vi "氨氮测量流程.vi"(11 "控制命令":T1(ring)) -> ()   [LabVIEW 2016, in "斯坦道氨氮.lvlib"]
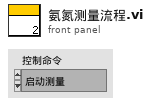
[diagram p1: front panel]
types:
  T1 = enum16{"启动测量", "标样核查", "零点核查", "跨度核查", "空白测试", "平行样测试", "加标回收", "空白校准", "标样校准", "初始化（清洗）", "停止测试", "仪器重启", "校时", "模式设置", "测量间隔设置"}
  T2 = cluster{"时间标识":timestamp, "设备":string, "日志信息":string, "流程参数":string}
  T3 = cluster{"站号":u16, "量程切换":enum32{"H", "L", "AUTO"}, "控制命令":enum16{"启动测量", "标样核查", "零点核查", "跨度核查", "空白测试", "平行样测试", "加标回收", "空白校准", "标样校准", "初始化（清洗）", "停止测试", "仪器重启", "校时", "模式设置", "测量间隔设置"}, "模式设置":enum16{"待机", "连续模式", "周期模式", "定点模式", "受控模式", "手动模式"}, "测量间隔":u16}
  T4 = cluster{"系统时间":timestamp, "工作状态":enum16{"空闲", "水样测试", "标样核查", "零点核查", "跨度核查", "空白测试", "平行样测试", "加标回收", "空白校准", "标样校准", "初始化（清洗）"}, "测量模式":enum16{"待机", "连续模式", "周期模式", "定点模式", "受控模式", "手动模式"}, "告警代码":u16, "故障代码":u16, "日志代码":u16, "软件版本":u16, "F0":sgl, "F1":sgl, "F2":sgl, "F3":sgl, "T":sgl, "H":sgl, "id":u16, "flowid":u16, "量程":u16, "总磷控温温度1":sgl, "营养盐控温温度2":sgl, "ADC":sgl}
  T5 = cluster{"水样测试量程模式":enum16{"H", "L", "AUTO"}, "空白核查量程模式":enum16{"H", "L", "AUTO"}, "跨度核查量程模式":enum16{"H", "L", "AUTO"}, "加标回收量程模式":enum16{"H", "L", "AUTO"}}
  T6 = enum16{"空闲", "水样测试", "标样核查", "零点核查", "跨度核查", "空白测试", "平行样测试", "加标回收", "空白校准", "标样校准", "初始化（清洗）"}
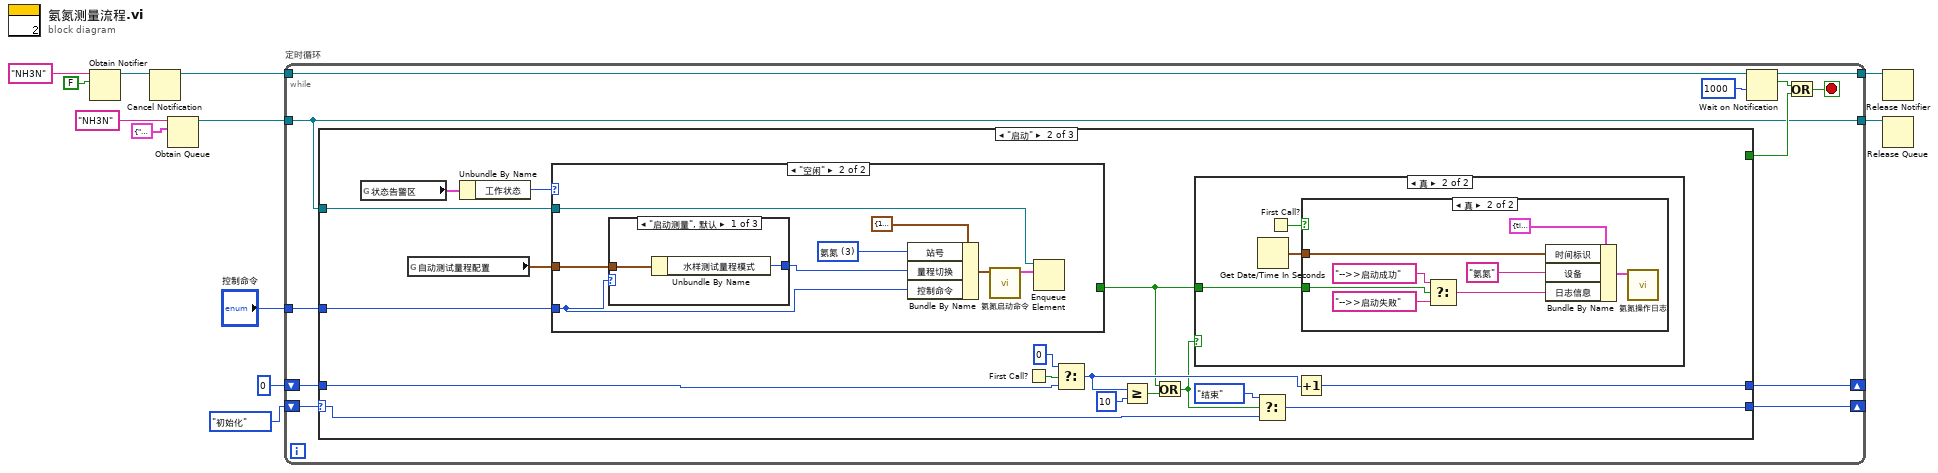
[diagram p0: block diagram]
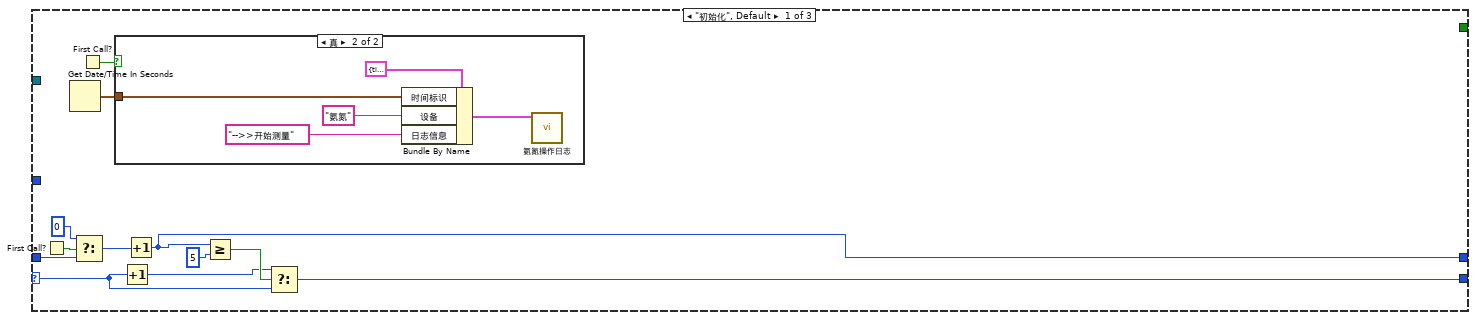
[diagram p2: hidden frame]
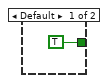
[diagram p6: hidden frame]
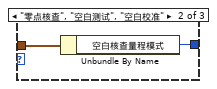
[diagram p7: hidden frame]
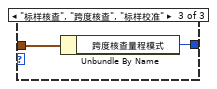
[diagram p8: hidden frame]
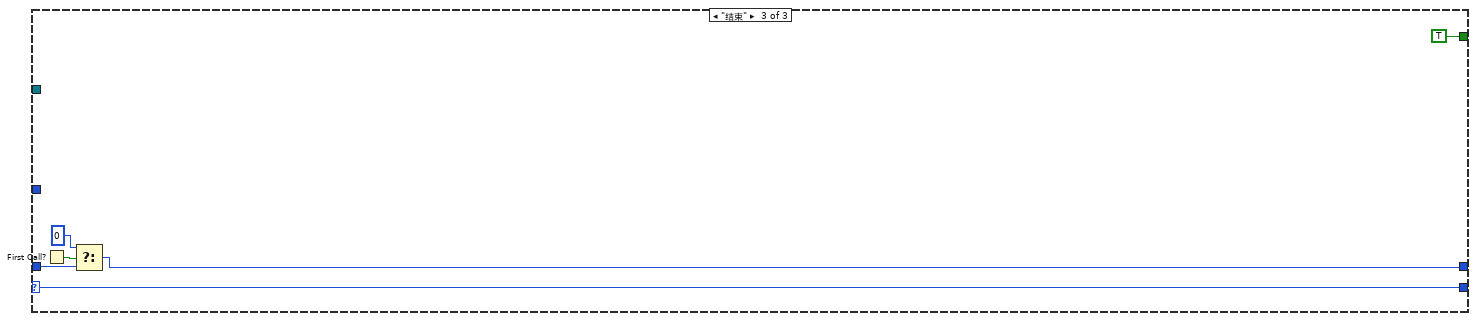
[diagram p9: hidden frame]
diagram:
  n1 = Obtain Notifier(name (unnamed)="NH3N" ("名称（未命名）"), notification data type=FALSE) -> (notifier out=w7:refnum<notifier>)  [unwired: 2 in, 2 out]
  n2 = Cancel Notification(0:w7) -> (8:w6:refnum<notifier>)  [unwired: 1 in, 2 out]
  n3 = Obtain Queue(name (unnamed)="NH3N" ("名称（未命名）"), element data type=cluster{"命令":string, "data":variant} {"命令"="", "data"=variant}) -> (queue out=w10:refnum<queue>)  [unwired: 3 in, 2 out]
  n4 = while "定时循环" {
    tunnel: w10 -> [w13]
    tunnel: w6 -> [w24]
    tunnel: "控制命令" -> [w19]
    shift-right: [w18] -> _
    shift-left: enum16{"初始化", "启动", "结束"}."初始化" -> [w20]
    shift-right: [w16] -> _
    shift-left: 0 -> [w17]
    tunnel: [w14] -> w2
    tunnel: [w13] -> w3
    stop <- w21 stop-if-true
    n5 = case shown="\"启动\"" w20 {
      selector: w20 -> [w26 w47 w90]
      tunnel: w19 -> [_ w58 _]
      tunnel: w13 -> [_ w57 _]
      tunnel: [w25 w48 w90] -> w18
      tunnel: w17 -> [w33 w52 w87]
      tunnel: [w30 w51 w86] -> w16
      tunnel: [_ _ TRUE] -> w15
      frame "初始化", Default {
        n6 = First Call?() -> (First Call?: T/F=w34:bool)
        n7 = Get Date/Time In Seconds() -> (seconds since 1Jan1904=w36:timestamp)
        n8 = Select(t=0, s=w34, f=w33) -> (s? t:f=w31:i32)
        n9 = First Call?() -> (First Call?: T/F=w35:bool)
        n10 = case shown="真" w35 {
          tunnel: w36 -> [_ w40]
          frame False {
          }
          frame True {
            n11 = Bundle By Name(cluster=T2 {"时间标识"=timestamp(0 s since 1904-01-01), "设备"="", "日志信息"="", "流程参数"=""} ("data in"), "时间标识"=w40, "设备"="氨氮", "日志信息"="-->>开始测量") -> (w41:T2)
            n12 = call "氨氮操作日志.vi"("data in"=w41) -> ()  [unwired: 11 in]
          }
        }
        n13 = Increment(x=w26) -> (x+1=w27:enum16{"初始化", "启动", "结束"})
        n14 = Increment(x=w31) -> (x+1=w30:i32)
        n15 = Greater Or Equal?(x=w30, y=5) -> (x >= y?=w28:bool)
        n16 = Select(t=w27, s=w28, f=w26) -> (s? t:f=w25:enum16{"初始化", "启动", "结束"})
      }
      frame "启动" {
        n17 = global read "VAR氨氮全局变量.vi" "状态告警区"() -> (w56:T4)
        n18 = global read "氨氮断电保存全局变量.vi" "自动测试量程配置"() -> (w42:T5)
        n19 = Unbundle By Name(w56) -> ("工作状态"=w55:T6)
        n20 = case shown="\"空闲\"" w55 {
          tunnel: w42 -> [_ w76]
          tunnel: w58 -> [_ w71]
          tunnel: w57 -> [_ w75]
          tunnel: [TRUE _] -> w43
          frame Default {
          }
          frame "空闲" {
            w74 = u16 3 items=["总磷"=1, "总氮"=2, "氨氮"=3] ("站号")
            n21 = case shown="\"启动测量\", 默认" w71 {
              tunnel: w76 -> [w80 w82 w84]
              tunnel: [w79 w81 w83] -> w78
              frame "启动测量", Default {
                n22 = Unbundle By Name(w80) -> ("水样测试量程模式"=w79:enum16{"H", "L", "AUTO"})
              }
              frame "零点核查", "空白测试", "空白校准" {
                n23 = Unbundle By Name(w82) -> ("空白核查量程模式"=w81:enum16{"H", "L", "AUTO"})
              }
              frame "标样核查", "跨度核查", "标样校准" {
                n24 = Unbundle By Name(w84) -> ("跨度核查量程模式"=w83:enum16{"H", "L", "AUTO"})
              }
            }
            n25 = Bundle By Name(cluster=T3 {"站号"=1, "量程切换"=enum."AUTO", "控制命令"=enum."启动测量", "模式设置"=enum."待机", "测量间隔"=0} ("参数"), "站号"=w74, "量程切换"=w78, "控制命令"=w71) -> (w72:T3)
            n26 = call "氨氮启动命令.vi"("参数"=w72) -> ("启动命令"=w77:cluster{"命令":string, "data":variant})  [unwired: 10 in]
            n27 = Enqueue Element(queue=w75, element=w77) -> ()  [unwired: 2 in, 3 out]
          }
        }
        n28 = First Call?() -> (First Call?: T/F=w54:bool)
        n29 = Select(t=0, s=w54, f=w52) -> (s? t:f=w50:i32)
        n30 = Greater Or Equal?(x=w50, y=10) -> (x >= y?=w46:bool)
        n31 = Or(x=w43, y=w46) -> (x .or. y?=w44:bool)
        n32 = case shown="真" w44 {
          tunnel: w43 -> [_ w59]
          frame False {
          }
          frame True {
            n33 = Get Date/Time In Seconds() -> (seconds since 1Jan1904=w60:timestamp)
            n34 = First Call?() -> (First Call?: T/F=w61:bool)
            n35 = case shown="真" w61 {
              tunnel: w60 -> [_ w68]
              tunnel: w59 -> [_ w65]
              frame False {
              }
              frame True {
                n36 = Select(t="-->>启动成功" ("日志信息"), s=w65, f="-->>启动失败" ("日志信息")) -> (s? t:f=w62:string)
                n37 = Bundle By Name(cluster=T2 {"时间标识"=timestamp(0 s since 1904-01-01), "设备"="", "日志信息"="", "流程参数"=""} ("data in"), "时间标识"=w68, "设备"="氨氮", "日志信息"=w62) -> (w69:T2)
                n38 = call "氨氮操作日志.vi"("data in"=w69) -> ()  [unwired: 11 in]
              }
            }
          }
        }
        n39 = Select(t=enum16{"初始化", "启动", "结束"}."结束", s=w44, f=w47) -> (s? t:f=w48:enum16{"初始化", "启动", "结束"})
        n40 = Increment(x=w50) -> (x+1=w51:i32)
      }
      frame "结束" {
        n41 = First Call?() -> (First Call?: T/F=w89:bool)
        n42 = Select(t=0, s=w89, f=w87) -> (s? t:f=w86:i32)
      }
    }
    n43 = Wait on Notification(notifier=w24, timeout in ms (-1)=1000 ("超时毫秒(-1)")) -> (notifier out=w14:refnum<notifier>, notification=w22:bool)  [unwired: 2 in, 2 out]
    n44 = Or(x=w22, y=w15) -> (x .or. y?=w21:bool)
  }
  n45 = Release Notifier(notifier=w2) -> ()  [unwired: 2 in, 3 out]
  n46 = Release Queue(queue=w3) -> ()  [unwired: 2 in, 3 out]
